vi "Decimate (multiple).vi"(8 "error in (no error)":errorcluster, 9 "Averaging (off)":bool, 10 "Decimation":i32, 11 "Multiple XY-data in":cluster{"X-array":dbl[], "Y-array":dbl[]}[](array[cluster]) {"Y-array" format="%.2p"; "X-array" format="%.2p"}) -> (0 "error out":errorcluster, 3 "Multiple XY-data out":cluster{"X-array":dbl[], "Y-array":dbl[]}[](array[cluster]) {"Y-array" format="%.2p"; "X-array" format="%.2p"})   [LabVIEW 2016, in "xy_utilities.lvlib"]
uses:
  xy_utilities.lvlib
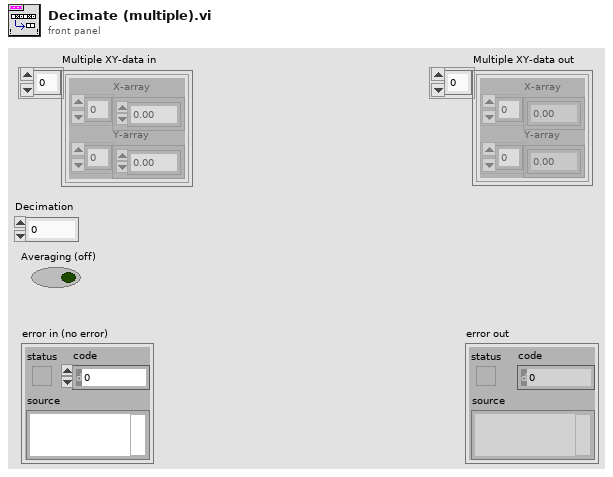
[diagram p1: front panel]
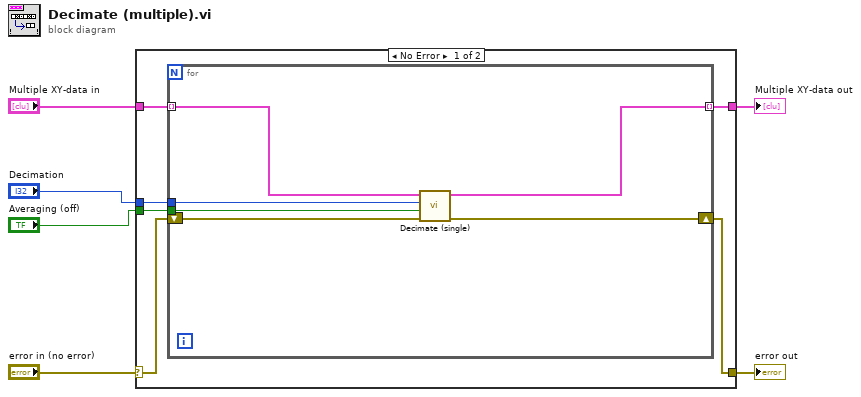
[diagram p0: block diagram]
diagram:
  n1 = case shown="No Error" "error in (no error)" {
    selector: "error in (no error)" -> [w10 w20]
    tunnel: "Multiple XY-data in" -> [w12 w19]
    tunnel: [w11 w19] -> w4
    tunnel: [w9 w20] -> w3
    tunnel: "Decimation" -> [w8 _]
    tunnel: "Averaging (off)" -> [w7 _]
    frame No Error {
      n2 = for {
        tunnel: w12 -> [w18] mode=indexing
        tunnel: [w17] -> w11 mode=indexing
        shift-right: [w15] -> w9
        shift-left: w10 -> [w16]
        tunnel: w8 -> [w14]
        tunnel: w7 -> [w13]
        n3 = call "Decimate (single).vi"("error in (no error)"=w16, "Averaging (off)"=w13, "Decimation (1)"=w14, "XY-data in"=w18) -> ("error out"=w15:errorcluster, "XY-data out"=w17:cluster{"X-array":dbl[], "Y-array":dbl[]})  [unwired: 6 in]
      }
    }
    frame Error {
    }
  }
  "error out" <- w3
  "Multiple XY-data out" <- w4
